vi "Main.vi"() -> ()   [LabVIEW 2013]
uses:
  Global.vi
panel:
  out "Error TCP_quad":errorcluster
  out "TCP_quad ID":refnum<k5>
  in  "Quadcopter":bool
  out "Trailers":bool[](array[boolean])
  out "Platooning Distance Scenario":dbl
  out "Distance2Master Scenario":dbl[](array[numeric])
  out "CurrentWP Final DarkGrey":i32
  out "Vref DarkGrey Final":dbl
  out "CurrentWP Final Grey":i32
  out "Vref Grey Final":dbl
  out "CurrentWP Final Black":i32
  out "Vref Black Final":dbl
  out "CurrentWP Final Blue":i32
  out "Vref Blue Final":dbl
  out "CurrentWP Final Red":i32
  out "Vref Red Final":dbl
  in  "Platooning Speed  Increment":dbl=1.25
  out "StopArrayOuter":i32[](array[numeric])
  out "StopArrayInner":i32[](array[numeric])
  out "PlatoonArray":i32[](array[numeric])
  out "Grey Truck Pose":sgl[](array[numeric])
  out "DarkGrey Truck Pose":dbl[](array[numeric])
  out "Current DarkGrey State":i32
  out "DarkGrey Trajectory WP Out":dbl[][](array[numeric])
  out "Red distance2Master DarkGrey":dbl
  out "DarkGrey dref":dbl
  out "Red distance2Master Grey":dbl
  out "Current Grey State":i32
  out "Grey Trajectory WP Out":dbl[][](array[numeric])
  out "Grey dref":dbl
  out "Change to state DarkGrey Scenario":i32
  out "Vref DarkGrey Scenario":dbl
  out "Change to state Grey Scenario":i32
  out "Vref Grey Scenario":dbl
  in  "ID DarkGrey":u8=5
  in  "ID Grey":u8=4
  in  "Change to state DarkGrey":i32(ring)=1 items=["Parking", "OuterLane", "InnerLane", "InnerRoad"]
  in  "Vref DarkGrey":dbl(slide) scale=0.0..1.5
  in  "Change to state Grey":i32(ring)=1 items=["Parking", "OuterLane", "InnerLane", "InnerRoad"]
  in  "Vref Grey":dbl(slide) scale=0.0..1.5
  out "X Grey":dbl
  out "Y  Grey":dbl
  out "Yaw  Grey":dbl
  out "X DarkGrey":dbl
  out "Y  DarkGrey":dbl
  out "Yaw  DarkGrey":dbl
  in  "ControllerGains DarkGrey":T1={"KPSteering"=1.0, "KDSteering"=0.0, "KPSpeed"=0.8, "KISpeed"=3.0, "KDSpeed"=0.2}
  out "Current state DarkGrey":i32(ring)=1 items=["Parking", "OuterLane", "InnerLane", "InnerRoad"]
  out "D2TL DarkGrey":dbl
  out "D2Master DarkGrey":dbl
  in  "With Trailer DarkGrey":bool
  out "Real Speed DarkGrey":dbl(knob) scale=0.0..2.0
  out "DarkGrey Speed":u8
  out "DarkGrey Steering":u8
  in  "ControllerGains Grey":T1={"KPSteering"=0.6, "KDSteering"=0.05, "KPSpeed"=0.8, "KISpeed"=3.0, "KDSpeed"=0.2}
  out "Current state Grey":i32(ring)=1 items=["Parking", "OuterLane", "InnerLane", "InnerRoad"]
  out "D2TL Grey":dbl
  out "D2Master Grey":dbl
  in  "With Trailer Grey":bool
  out "Real Speed Grey":dbl(knob) scale=0.0..2.0
  out "Grey Speed":u8
  out "Grey Steering":u8
  out "COM  DarkGrey":T2
  out "COM  Grey":T2
  in  "DarkGrey ID":u8=9
  in  "Grey ID":u8=8
  in  "Port DarkGrey":u16=9006
  in  "Port Grey":u16=9005
  in  "QTM ID DarkGrey":i32=3
  in  "QTM ID Grey":i32=5
  out "Vref":dbl[](array[numeric])
  out "bytes written 3":i32
  out "bytes written 2":i32
  out "ScenarioString":string
  out "red dref":dbl
  out "real distance2master red":dbl
  in  "ControllerGains Black":T1={"KPSteering"=0.9, "KDSteering"=0.05, "KPSpeed"=1.0, "KISpeed"=3.0, "KDSpeed"=0.2}
  in  "ControllerGains Blue":T1={"KPSteering"=1.0, "KDSteering"=0.05, "KPSpeed"=0.8, "KISpeed"=3.0, "KDSpeed"=0.2}
  out "Version":i32
  in  "Visualizer":bool
  out "Iter":i32
  out "NRoads":i32
  out "TL Outer Select":bool
  out "TL Inner Select":bool
  out "Error TCP":errorcluster
  out "TCP ID":refnum<k5>
  out "NTrucks":i32
  out "CurrentWP":i32[](array[numeric])
  out "Change to state Red Scenario":i32
  out "Vref Red Scenario":dbl
  out "Change to state Blue Scenario":i32
  out "Vref Blue Scenario":dbl
  out "Change to state Black Scenario":i32
  out "Vref Black Scenario":dbl
  out "Ignore":bool
  out "Current state Red":i32(ring)=1 items=["Parking", "OuterLane", "InnerLane", "InnerRoad"]
  out "Current state Blue":i32(ring)=1 items=["Parking", "OuterLane", "InnerLane", "InnerRoad"]
  out "Current state Black":i32(ring)=1 items=["Parking", "OuterLane", "InnerLane", "InnerRoad"]
  in  "Tab Control":enum32{"Pedro Lima", "João Pedro Alvito"}(tab)
  in  "Scenario Selection PL":u32(ring) items=["Manual", "1 catch up 1", "1 catch up 2", "2 catch up 1", "1 catch up 1 from other road", "1 catch up 1 but master exits", "1 diferent mass catch up 2 without overtake", "1 different mass catch up 2 with overtake", "1 catch up 2 but middle leaves"]
  out "Info PL":string
  out "length":i32
  in  "Bridge":bool
  in  "Scenario Selection JPA":u32(ring) items=["Manual", "Simple traffic lights", "Simple anti-platoon", "Mixture", "Time Decision", "Timed Control with Platoon", "Anti-platoon"]
  out "Info JP":string
  out "X Red":dbl
  out "Y  Red":dbl
  out "Yaw  Red":dbl
  out "X Black":dbl
  out "Y Black":dbl
  out "Yaw Black":dbl
  out "Yaw Blue":dbl
  out "Y Blue":dbl
  out "X Blue":dbl
  out "D2TL Red":dbl
  out "D2TL Black":dbl
  out "D2TL Blue":dbl
  out "D2Master Red":dbl
  out "D2Master Black":dbl
  out "D2Master Blue":dbl
  out "Outer Red":bool
  out "Inner Green":bool
  out "Inner Red":bool
  out "Outer Green":bool
  out "D2TLFinal":dbl[](array[numeric])
  out "Truck Dimensions":dbl[](array[numeric])
  out "Traffic Lights":T3
  in  "Stop Button Inner":bool
  in  "Traffic Light Position Inner Lane":i32=23
  out "CurrentState":i32[](array[numeric])
  out "Real Speed Red":dbl(knob) scale=0.0..2.0
  out "Real Speed Black":dbl(knob) scale=0.0..2.0
  in  "Stop Button Outer":bool
  in  "Traffic Light Position Outer Lane":i32=27
  out "InnerRoad":T4
  out "Distance to Master":dbl[](array[numeric])
  out "Blue dref":dbl
  out "Blue distance2master blue":dbl
  out "black dref":dbl
  out "Red distance2Master black":dbl
  out "Red Trajectory WP Out":dbl[][](array[numeric])
  out "Blue Trajectory WP Out":dbl[][](array[numeric])
  out "Black Trajectory WP Out":dbl[][](array[numeric])
  in  "Change to state Black":i32(ring)=1 items=["Parking", "OuterLane", "InnerLane", "InnerRoad"]
  in  "Change to state Red":i32(ring)=1 items=["Parking", "OuterLane", "InnerLane", "InnerRoad"]
  out "Trajectory Network":T5(array[cluster])
  out "InnerLane":T4
  out "OuterLane":T4
  out "Current Red State":i32
  out "Current Black State":i32
  out "Current Blue State":i32
  in  "Change to state Blue":i32(ring)=1 items=["Parking", "OuterLane", "InnerLane", "InnerRoad"]
  out "Trucks Poses":dbl[][](array[numeric])
  out "Total Platooning Distance":dbl[](array[numeric])
  in  "With Trailer Red":bool
  in  "With Trailer  Black":bool
  in  "With Trailer Blue":bool
  in  "QTM ID Red":i32=4
  in  "QTM ID Blue":i32=2
  in  "QTM ID Black":i32=1
  in  "ID Black":u8=2
  in  "ID Red":u8=3
  in  "ID Blue":u8=1
  out "COM  Black":T2
  out "COM  Red":T2
  out "COM Blue":T2
  in  "Platooning Distance":dbl=0.3
  out "Distance2Master":dbl[](array[numeric])
  out "Real Speed Blue":dbl(knob) scale=0.0..2.0
  in  "Set MasterID":i32(ring) items=["None", "Blue Truck", "Black Truck", "Red Truck", "Grey Truck", "DarkGrey Truck"]
  in  "Vref Black":dbl(slide) scale=0.0..1.5
  in  "Vref Blue":dbl(slide) scale=0.0..1.5
  in  "Vref Red":dbl(slide) scale=0.0..1.5
  out "Red Truck Pose":dbl[](array[numeric])
  out "Blue Truck Pose":dbl[](array[numeric])
  out "Black Truck Pose":dbl[](array[numeric])
  out "Red Speed":u8
  out "Red Steering":u8
  in  "stop":bool
  out "Blue Speed":u8
  out "Blue Steering":u8
  in  "Port Blue":u16=9002
  in  "Blue ID":u8=10
  in  "Port":u16=22222 min=22222
  in  "Address":string="130.237.50.220"
  in  "Port Red":u16=9004
  in  "Red ID":u8=7
  out "Black Speed":u8
  out "Black Steering":u8
  in  "Port Black":u16=9003
  in  "Black ID":u8=14
  in  "ControllerGains Red":T1={"KPSteering"=1.0, "KDSteering"=0.05, "KPSpeed"=0.8, "KISpeed"=3.0, "KDSpeed"=0.2}
types:
  T1 = cluster{"KPSteering":dbl, "KDSteering":dbl, "KPSpeed":dbl, "KISpeed":dbl, "KDSpeed":dbl}
  T2 = cluster{"Truck ID":u8, "connection ID":refnum<k5>}
  T3 = cluster{"Stop Button Outer":bool, "Stop WP Outer Lane":dbl, "Stop Button Inner":bool, "Stop WP Inner Lane ":dbl}
  T4 = cluster{"all rows":dbl[][], "all rows":dbl[][], "Array":i32[]}
  T5 = cluster{"Trajectory WP":dbl[][], "Distances LUT":dbl[][], "Trajectory length":i32[]}[]
  T6 = cluster{"pose":dbl[], "totalerror_v":dbl, "erroSteering":dbl, "ActualTime":dbl, "ActualTime 2":dbl}
  T7 = cluster{"all rows":dbl[][], "all rows":dbl[][], "Array":i32[]}[]
  T8 = cluster{"Trajectory WP":dbl[][], "Distances LUT":dbl[][], "Trajectory length":i32[]}
  T9 = cluster{"Vref Black":dbl, "Change to state Black":i32, "Vref Blue":dbl, "Change to state Blue":i32, "Vref Red":dbl, "Change to state Red":i32, "Vref Grey":dbl, "Change to state Grey":i32, "Vref DarkGrey":dbl, "Change to state DarkGrey":i32, "With Trailer Blue":bool, "With Trailer  Black":bool, "With Trailer Red":bool, "With Trailer Grey":bool, "With Trailer DarkGrey":bool, "Platooning Distance":dbl, "CurrentWP":i32[], "Distance to Master":dbl[], "D2TLFinal":dbl[], "CurrentState":i32[], "Trajectory Network":cluster{"Trajectory WP":dbl[][], "Distances LUT":dbl[][], "Trajectory length":i32[]}[]}
  T10 = cluster{"Vref_Black":dbl, "Change_to_state_Black":i32, "Vref_Blue":dbl, "Change_to_state_Blue":i32, "Vref_Red":dbl, "Change_to_state_Red":i32, "Vref_Grey":dbl, "Change_to_state_Grey":i32, "Vref_DarkGrey":dbl, "Change_to_state_DarkGrey":i32, "With_Trailer_Blue":bool, "With_Trailer_Black":bool, "With_Trailer_Red":bool, "With_Trailer_Grey":bool, "With_Trailer_DarkGrey":bool, "Platooning_Distance":dbl, "CurrentWP":i32[], "Distance2Master":dbl[], "d2TL":dbl[], "CurrentState":i32[], "TrajectoryNetwork":cluster{"TrajectoryWP":dbl[][], "DistancesLUT":dbl[][], "TrajectoryLength":i32[]}[]}
  T11 = cluster{"Stop Button Outer":bool, "Traffic Light Position Outer Lane":i32, "Stop Button Inner":bool, "Traffic Light Position Inner Lane":i32}
  T12 = cluster{"pose":dbl[], "totalerror_v":dbl, "erroSteering":dbl, "ActualTime":dbl, "error_v":dbl}
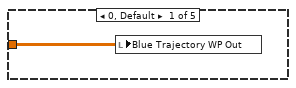
[diagram p5: hidden frame]
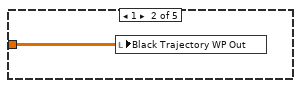
[diagram p6: hidden frame]
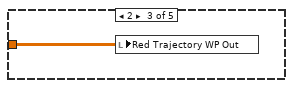
[diagram p7: hidden frame]
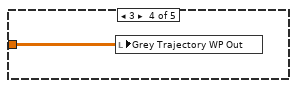
[diagram p8: hidden frame]
diagram:
  n1 = flat-sequence {
    frame #0 {
      n2 = flat-sequence {
        frame #0 {
          # "Initializations"
          n3 = Build Array(0 ("element"), 0 ("element"), 0 ("element"), 0 ("element"), 0 ("element")) -> (w78:i32[])
          "CurrentState" <- w78
          n4 = Build Array(0 ("element"), 0 ("element"), 0 ("element"), 0 ("element"), 0 ("element")) -> (→"CurrentWP":i32[])
          n5 = global write "Global.vi" "Transition WP"(i32[][] [[-1, -1, -1, -1], [-1, -1, -1, -1], [-1, -1, 5, 1], [-1, -1, 50, 25]] ("Transition WP")) -> ()
          n6 = global write "Global.vi" "RealSpeed"(dbl[] [] ("RealSpeed")) -> ()
          n7 = Build Array("Tab Control", "Scenario Selection PL", "Scenario Selection JPA") -> (w59:u32[])
          n8 = global write "Global.vi" "ScenarioArray"(w59) -> ()
          n9 = Array Size(array=w78) -> (size(s)=→"NTrucks":i32)
          n10 = local write "Set MasterID"(0 ("MasterID")) -> ()
          n11 = global write "Global.vi" "IsOvertaking"(FALSE ("IsOvertaking")) -> ()
          n12 = Index Array(array=w59, index=0) -> (element=w60:u32)
          n13 = global write "Global.vi" "Positioned"(FALSE ("FirstTime")) -> ()
          n14 = global write "Global.vi" "MasterID"(0 ("MasterID")) -> ()
          n15 = Increment(x=w60) -> (x+1=w61:u32)
          n16 = global write "Global.vi" "stop"(FALSE ("stop")) -> ()
          n17 = Index Array(array=w59, index=w61) -> (element=w62:u32)
          n18 = global write "Global.vi" "TL  Inner"(FALSE ("TL  Inner")) -> ()
          n19 = global write "Global.vi" "TL Outer"(FALSE ("TL Outer")) -> ()
          n20 = global write "Global.vi" "Lap Counter"(0 ("Lap Counter")) -> ()
          n21 = global write "Global.vi" "FirstTime"(TRUE ("FirstTime")) -> ()
          n22 = Not Equal To 0?(x=w62) -> (x != 0?=→"Ignore":bool)
          n23 = global write "Global.vi" "SetMasterID"(0 ("MasterID")) -> ()
          "ScenarioString" <- " " ("ScenarioString")
          "Vref" <- dbl[] [] ("RealSpeed")
        }
      }
      n24 = flat-sequence {
        frame #0 {
          n25 = local read "Tab Control"() -> (w2:enum32{"Pedro Lima", "João Pedro Alvito"})
          n26 = call "GetVersion.vi"() -> ("number"=→"Version":i32)
          n27 = Not Equal To 0?(x=w2) -> (x != 0?=w1:bool)
          n28 = local read "Version"() -> (w7:i32)
          n29 = local read "Version"() -> (w8:i32)
          n30 = local read "Version"() -> (w9:i32)
          n31 = local read "Version"() -> (w10:i32)
          n32 = local read "Version"() -> (w12:i32)
          n33 = local read "Version"() -> (w14:i32)
          n34 = local read "Version"() -> (w6:i32)
          n35 = local read "Version"() -> (w13:i32)
          n36 = call "CreatePath.vi"("Matlab Version"=w7, "filename"="OuterLaneBridgeLUT.txt") -> ("FinalPath"=w20:path)
          n37 = call "CreatePath.vi"("Matlab Version"=w8, "filename"="OuterLaneLUT.txt") -> ("FinalPath"=w22:path)
          n38 = call "CreatePath.vi"("Matlab Version"=w9, "filename"="OuterLaneBridge.txt") -> ("FinalPath"=w24:path)
          n39 = call "CreatePath.vi"("Matlab Version"=w10, "filename"="OuterLane.txt") -> ("FinalPath"=w26:path)
          n40 = call "CreatePath.vi"("Matlab Version"=w12, "filename"="InnerLaneBridgeLUT.txt") -> ("FinalPath"=w34:path)
          n41 = call "CreatePath.vi"("Matlab Version"=w14, "filename"="InnerLaneLUT.txt") -> ("FinalPath"=w33:path)
          n42 = call "CreatePath.vi"("Matlab Version"=w6, "filename"="InnerLaneBridge.txt") -> ("FinalPath"=w30:path)
          n43 = call "CreatePath.vi"("Matlab Version"=w13, "filename"="InnerLane.txt") -> ("FinalPath"=w28:path)
          n44 = local read "Version"() -> (w11:i32)
          n45 = local read "Version"() -> (w15:i32)
          n46 = And(x="Bridge", y=w1) -> (x .and. y?=w4:bool)
          n47 = call "CreatePath.vi"("Matlab Version"=w11, "filename"="InnerRoadLUT.txt") -> ("FinalPath"=w16:path)
          n48 = call "CreatePath.vi"("Matlab Version"=w15, "filename"="InnerRoad.txt") -> ("FinalPath"=w18:path)
          n49 = Select(t=w20, s=w4, f=w22) -> (s? t:f=w41:path)
          n50 = Select(t=w24, s=w4, f=w26) -> (s? t:f=w40:path)
          n51 = Select(t=w34, s=w4, f=w33) -> (s? t:f=w38:path)
          n52 = Select(t=w30, s=w4, f=w28) -> (s? t:f=w39:path)
          n53 = call "ReadFromFile.vi"("Trajectory Path File"=w40, "Trajectory Distances LUT"=w41) -> ("Trajectory Data"=w45:T4)  [unwired: 1 in]
          "OuterLane" <- w45
          n54 = call "ReadFromFile.vi"("Trajectory Path File"=w18, "Trajectory Distances LUT"=w16) -> ("Trajectory Data"=w42:T4)  [unwired: 1 in]
          "InnerRoad" <- w42
          n55 = call "ReadFromFile.vi"("Trajectory Path File"=w39, "Trajectory Distances LUT"=w38) -> ("Trajectory Data"=w44:T4)  [unwired: 1 in]
          "InnerLane" <- w44
          n56 = Build Array(T4 {"all rows"=[], "all rows"=[], "Array"=[]} ("element"), w45, w44, w42) -> (w37:T7)
          "Trajectory Network" <- w37
          n57 = Array Size(array=w37) -> (size(s)=→"NRoads":i32)
        }
      }
      n58 = flat-sequence {
        frame #0 {
          n59 = call "CreateConnection.vi"("Truck ID"="DarkGrey ID", "Port number\nactuators"="Port DarkGrey") -> ("COM data"=→"COM  DarkGrey":T2)  [unwired: 1 in]
          n60 = call "CreateConnection.vi"("Truck ID"="Red ID", "Port number\nactuators"="Port Red") -> ("COM data"=→"COM  Red":T2)  [unwired: 1 in]
          n61 = call "CreateConnection.vi"("Truck ID"="Black ID", "Port number\nactuators"="Port Black") -> ("COM data"=→"COM  Black":T2)  [unwired: 1 in]
          n62 = call "CreateConnection.vi"("Truck ID"="Blue ID", "Port number\nactuators"="Port Blue") -> ("COM data"=→"COM Blue":T2)  [unwired: 1 in]
          n63 = call "CreateConnection.vi"("Truck ID"="Grey ID", "Port number\nactuators"="Port Grey") -> ("COM data"=→"COM  Grey":T2)  [unwired: 1 in]
        }
      }
    }
    frame #1 {
      n64 = local read "Visualizer"() -> (w98:bool)
      n65 = local read "Quadcopter"() -> (w97:bool)
      n66 = case shown="True" w98 {
        frame False {
        }
        frame True {
          n67 = flat-sequence {
            frame #0 {
              n68 = local read "Trajectory Network"() -> (w109:T5)
              n69 = Index Array(array=w109) -> (element #2=w110:T8, element #3=w111:T8, element #4=w112:T8)  [unwired: 4 in, 1 out]
              n70 = Unbundle By Name(w110) -> ("Trajectory length"=w116:i32[], "Trajectory WP"=w124:dbl[][])
              n71 = Unbundle By Name(w111) -> ("Trajectory length"=w120:i32[], "Trajectory WP"=w125:dbl[][])
              n72 = Unbundle By Name(w112) -> ("Trajectory length"=w121:i32[], "Trajectory WP"=w126:dbl[][])
              n73 = Index Array(array=w116, index=0) -> (element=w127:i32)
              n74 = Index Array(array=w120, index=0) -> (element=w129:i32)
              n75 = Index Array(array=w121, index=0) -> (element=w131:i32)
              n76 = local read "NRoads"() -> (w138:i32)
              n77 = Multiply(x=w127, y=2) -> (x*y=w122:i32)
              n78 = Multiply(x=w129, y=2) -> (x*y=w123:i32)
              n79 = Multiply(x=w131, y=2) -> (x*y=w103:i32)
              n80 = Reshape Array(w124, w122) -> (w128:dbl[])
              n81 = Reshape Array(w125, w123) -> (w130:dbl[])
              n82 = Reshape Array(w126, w103) -> (w132:dbl[])
              n83 = Subtract(x=w138, y=1) -> (x-y=w139:i32)
              n84 = Build Array (concatenate)(w139, w127, w128, w129, w130, w131, w132) -> (w106:dbl[])
              n85 = To Double Precision Float(number=w106) -> (double precision float=w107:dbl[])
              n86 = Type Cast(x=w107) -> (*(type *) &x=w108:string)  [unwired: 1 in]
              n87 = call <vilib>:"TCP Listen.vi"("timeout ms (wait forever: -1)"=-1, "port"=u16 55000 ("remote port or service name")) -> ("error out"=w134:errorcluster, "connection ID"=w133:refnum<k5>)  [unwired: 5 in, 3 out]
              n88 = TCP Write(connection ID=w133, data in=w108, error in (no error)=w134) -> (connection ID out=→"TCP ID":refnum<k5>, error out=→"Error TCP":errorcluster)  [unwired: 1 in, 1 out]
            }
            frame #1 {
              n89 = local read "Bridge"() -> (w141:bool)
              n90 = Boolean To (0,1)(Boolean=w141) -> (0, 1=w140:i16)
              n91 = global read "Global.vi" "ScenarioArray"() -> (w143:u32[])
              n92 = local read "NTrucks"() -> (w142:i32)
              n93 = Build Array (concatenate)(w143, w142, w140) -> (w145:u32[])
              n94 = To Double Precision Float(number=w145) -> (double precision float=w144:dbl[])
              n95 = Type Cast(x=w144) -> (*(type *) &x=w146:string)  [unwired: 1 in]
              n96 = local read "Error TCP"() -> (w148:errorcluster)
              n97 = local read "TCP ID"() -> (w147:refnum<k5>)
              n98 = TCP Write(connection ID=w147, data in=w146, error in (no error)=w148) -> (connection ID out=w150:refnum<k5>, error out=w149:errorcluster)  [unwired: 1 in, 1 out]
              n99 = local write "TCP ID"(w150) -> ()
              n100 = local write "Error TCP"(w149) -> ()
            }
          }
        }
      }
      n101 = case shown="True" w97 {
        frame False {
        }
        frame True {
          n102 = call <vilib>:"TCP Listen.vi"("timeout ms (wait forever: -1)"=-1, "port"=u16 56999 ("remote port or service name")) -> ("error out"=→"Error TCP_quad":errorcluster, "connection ID"=→"TCP_quad ID":refnum<k5>)  [unwired: 5 in, 3 out]
        }
      }
    }
    frame #2 {
      n103 = while {
        i -> [w151]
        stop <- "stop" stop-if-true
        n104 = flat-sequence {
          frame #0 {
            n105 = call "GetPose.vi"("port"="Port", "address"="Address", "QTM ID"="QTM ID Blue") -> ("Pose"=w164:dbl[])  [unwired: 8 in]
            "Blue Truck Pose" <- w164
            n106 = call "GetPose.vi"("port"="Port", "address"="Address", "QTM ID"="QTM ID Grey") -> ("Pose"=w160:dbl[])  [unwired: 8 in]
            "Grey Truck Pose" <- w160
            n107 = call "GetPose.vi"("port"="Port", "address"="Address", "QTM ID"="QTM ID DarkGrey") -> ("Pose"=w158:dbl[])  [unwired: 8 in]
            "DarkGrey Truck Pose" <- w158
            n108 = call "GetPose.vi"("port"="Port", "address"="Address", "QTM ID"="QTM ID Black") -> ("Pose"=w162:dbl[])  [unwired: 8 in]
            "Black Truck Pose" <- w162
            n109 = call "GetPose.vi"("port"="Port", "address"="Address", "QTM ID"="QTM ID Red") -> ("Pose"=w156:dbl[])  [unwired: 8 in]
            "Red Truck Pose" <- w156
            n110 = Build Array(w164, w162, w156, w160, w158) -> (→"Trucks Poses":dbl[][])
            n111 = Index Array(array=w164) -> (element #1=→"X Blue":dbl, element #2=→"Y Blue":dbl, element #3=→"Yaw Blue":dbl)  [unwired: 3 in]
            n112 = Index Array(array=w162) -> (element #1=→"X Black":dbl, element #2=→"Y Black":dbl, element #3=→"Yaw Black":dbl)  [unwired: 3 in]
            n113 = Index Array(array=w160) -> (element #1=→"X Grey":dbl, element #2=→"Y  Grey":dbl, element #3=→"Yaw  Grey":dbl)  [unwired: 3 in]
            n114 = Index Array(array=w158) -> (element #1=→"X DarkGrey":dbl, element #2=→"Y  DarkGrey":dbl, element #3=→"Yaw  DarkGrey":dbl)  [unwired: 3 in]
            n115 = Index Array(array=w156) -> (element #1=→"X Red":dbl, element #2=→"Y  Red":dbl, element #3=→"Yaw  Red":dbl)  [unwired: 3 in]
          }
          frame #1 {
            w193 = 0.5 ("t")
            w194 = 1.3 ("t")
            n116 = local read "Trajectory Network"() -> (w207:T5)
            n117 = local read "Distance to Master"() -> (w210:dbl[])
            n118 = local read "CurrentState"() -> (w208:i32[])
            n119 = local read "CurrentWP"() -> (w211:i32[])
            n120 = local read "D2TLFinal"() -> (w209:dbl[])
            n121 = Bundle("Vref Black"="Vref Black", "Change to state Black"="Change to state Black", "Vref Blue"="Vref Blue", "Change to state Blue"="Change to state Blue", "Vref Red"="Vref Red", "Change to state Red"="Change to state Red", "Vref Grey"="Vref Grey", "Change to state Grey"="Change to state Grey", "Vref DarkGrey"="Vref DarkGrey", "Change to state DarkGrey"="Change to state DarkGrey", "With Trailer Blue"="With Trailer Blue", "With Trailer  Black"="With Trailer  Black", "With Trailer Red"="With Trailer Red", "With Trailer Grey"="With Trailer Grey", "With Trailer DarkGrey"="With Trailer DarkGrey", "Platooning Distance"="Platooning Distance", "CurrentWP"=w211, "Distance to Master"=w210, "D2TLFinal"=w209, "CurrentState"=w208, "Trajectory Network"=w207) -> (w199:T9)  [unwired: 1 in]
            n122 = call "ScenarioScript.vi"("Control In"=w199) -> ("Control Out"=w219:T10, "String"=w206:string)
            "Info PL" <- w206
            "Info JP" <- w206
            n123 = local write "ScenarioString"(w206) -> ()
            n124 = Unbundle By Name(w219) -> ("Vref_Black"=→"Vref Black Scenario":dbl, "Change_to_state_Black"=→"Change to state Black Scenario":i32, "Vref_Blue"=→"Vref Blue Scenario":dbl, "Change_to_state_Blue"=→"Change to state Blue Scenario":i32, "Vref_Red"=→"Vref Red Scenario":dbl, "Change_to_state_Red"=→"Change to state Red Scenario":i32, "Vref_Grey"=→"Vref Grey Scenario":dbl, "Change_to_state_Grey"=→"Change to state Grey Scenario":i32, "Vref_DarkGrey"=→"Vref DarkGrey Scenario":dbl, "Change_to_state_DarkGrey"=→"Change to state DarkGrey Scenario":i32, "With_Trailer_Blue"=w187:bool, "With_Trailer_Black"=w186:bool, "With_Trailer_Red"=w185:bool, "With_Trailer_Grey"=w184:bool, "With_Trailer_DarkGrey"=w183:bool, "Platooning_Distance"=w213:dbl, "Distance2Master"=w190:dbl[])
            "Platooning Distance Scenario" <- w213
            n125 = Select(t=w194, s=w187, f=w193) -> (s? t:f=w230:dbl)
            n126 = Select(t=w194, s=w186, f=w193) -> (s? t:f=w231:dbl)
            n127 = Select(t=w194, s=w185, f=w193) -> (s? t:f=w232:dbl)
            n128 = Select(t=w194, s=w184, f=w193) -> (s? t:f=w192:dbl)
            n129 = Select(t=w194, s=w183, f=w193) -> (s? t:f=w191:dbl)
            n130 = Build Array(w187, w186, w185, w184, w183) -> (→"Trailers":bool[])
            n131 = Build Array(w230, w231, w232, w192, w191) -> (w189:dbl[])
            "Truck Dimensions" <- w189
            n132 = Add(x=w189, y=w213) -> (x+y=→"Total Platooning Distance":dbl[])
            n133 = Add(x=w190, y=w189) -> (x+y=→"Distance2Master Scenario":dbl[])
          }
          frame #2 {
            n134 = local read "Change to state DarkGrey Scenario"() -> (w281:i32)
            n135 = local read "Change to state Black Scenario"() -> (w304:i32)
            n136 = local read "Change to state Grey Scenario"() -> (w294:i32)
            n137 = local read "Change to state Blue Scenario"() -> (w303:i32)
            n138 = local read "Platooning Speed  Increment"() -> (w264:dbl)
            n139 = local read "Platooning Speed  Increment"() -> (w268:dbl)
            n140 = local read "Platooning Speed  Increment"() -> (w267:dbl)
            n141 = local read "Change to state Red Scenario"() -> (w305:i32)
            n142 = local read "Platooning Speed  Increment"() -> (w266:dbl)
            n143 = local read "Platooning Speed  Increment"() -> (w265:dbl)
            n144 = local read "Total Platooning Distance"() -> (w314:dbl[])
            n145 = local read "Distance2Master Scenario"() -> (w328:dbl[])
            n146 = local read "Total Platooning Distance"() -> (w290:dbl[])
            n147 = local read "Distance2Master Scenario"() -> (w286:dbl[])
            n148 = local read "Total Platooning Distance"() -> (w277:dbl[])
            n149 = local read "Distance2Master Scenario"() -> (w273:dbl[])
            n150 = local read "Total Platooning Distance"() -> (w330:dbl[])
            n151 = local read "Distance2Master Scenario"() -> (w329:dbl[])
            n152 = local read "Total Platooning Distance"() -> (w318:dbl[])
            n153 = local read "Distance2Master Scenario"() -> (w319:dbl[])
            n154 = local read "Vref DarkGrey Scenario"() -> (w254:dbl)
            n155 = local read "Real Speed DarkGrey"() -> (w269:dbl)
            n156 = local read "Trajectory Network"() -> (w316:T5)
            n157 = local read "Trajectory Network"() -> (w288:T5)
            n158 = local read "Trajectory Network"() -> (w275:T5)
            n159 = local read "Trajectory Network"() -> (w335:T5)
            n160 = local read "Trajectory Network"() -> (w321:T5)
            n161 = local read "Vref Black Scenario"() -> (w256:dbl)
            n162 = local read "Vref Grey Scenario"() -> (w255:dbl)
            n163 = local read "Vref Red Scenario"() -> (w258:dbl)
            n164 = local read "Vref Blue Scenario"() -> (w257:dbl)
            n165 = local read "Real Speed Black"() -> (w327:dbl)
            n166 = local read "Real Speed Blue"() -> (w339:dbl)
            n167 = local read "Real Speed Grey"() -> (w270:dbl)
            n168 = local read "Real Speed Red"() -> (w326:dbl)
            n169 = local read "PlatoonArray"() -> (w236:i32[])
            n170 = local read "Traffic Lights"() -> (w322:T3)
            n171 = local read "PlatoonArray"() -> (w235:i32[])
            n172 = local read "Traffic Lights"() -> (w287:T3)
            n173 = local read "PlatoonArray"() -> (w234:i32[])
            n174 = local read "Traffic Lights"() -> (w274:T3)
            n175 = local read "PlatoonArray"() -> (w238:i32[])
            n176 = local read "Traffic Lights"() -> (w323:T3)
            n177 = local read "PlatoonArray"() -> (w237:i32[])
            n178 = local read "Traffic Lights"() -> (w324:T3)
            n179 = local read "Trucks Poses"() -> (w315:dbl[][])
            n180 = local read "Trucks Poses"() -> (w289:dbl[][])
            n181 = local read "Trucks Poses"() -> (w276:dbl[][])
            n182 = local read "Trucks Poses"() -> (w333:dbl[][])
            n183 = local read "Trucks Poses"() -> (w331:dbl[][])
            n184 = local read "CurrentState"() -> (w312:i32[])
            n185 = local read "Set MasterID"() -> (w261:i32)
            n186 = local read "CurrentState"() -> (w292:i32[])
            n187 = local read "Set MasterID"() -> (w262:i32)
            n188 = local read "CurrentState"() -> (w279:i32[])
            n189 = local read "Set MasterID"() -> (w263:i32)
            n190 = local read "CurrentState"() -> (w325:i32[])
            n191 = local read "Set MasterID"() -> (w259:i32)
            n192 = local read "CurrentState"() -> (w317:i32[])
            n193 = local read "Set MasterID"() -> (w260:i32)
            n194 = local read "ID DarkGrey"() -> (w278:u8)
            n195 = local read "CurrentWP"() -> (w251:i32[])
            n196 = local read "CurrentWP"() -> (w250:i32[])
            n197 = local read "CurrentWP"() -> (w249:i32[])
            n198 = local read "CurrentWP"() -> (w253:i32[])
            n199 = local read "CurrentWP"() -> (w252:i32[])
            n200 = local read "D2TLFinal"() -> (w309:dbl[])
            n201 = local read "D2TLFinal"() -> (w293:dbl[])
            n202 = local read "D2TLFinal"() -> (w280:dbl[])
            n203 = local read "D2TLFinal"() -> (w311:dbl[])
            n204 = local read "D2TLFinal"() -> (w310:dbl[])
            n205 = local read "ID Black"() -> (w313:u8)
            n206 = local read "ID Grey"() -> (w291:u8)
            n207 = local read "ID Blue"() -> (w320:u8)
            n208 = local read "ID Red"() -> (w334:u8)
            n209 = call "DecisionMaker.vi"("Trajectory Network"=w316, "Change to state"=w304, "Vref"=w256, "K"=w264, "Platooning distances"=w314, "Current State In"=w312, "Set MasterID"=w261, "Current WP In"=w251, "MyID"=w313, "Distance2Master"=w328, "PlatoonArray"=w236, "Traffic Lights"=w322, "Trucks Poses"=w315, "d2TLFinal"=w309) -> ("d"=→"Red distance2Master black":dbl, "dref"=→"black dref":dbl, "Current State Out"=→"Current Black State" →"Current state Black":i32, "VrefOut"=→"Vref Black Final":dbl, "CurrentWPOut"=→"CurrentWP Final Black":i32, "Trajectory WP Out"=→"Black Trajectory WP Out":dbl[][])  [unwired: 8 in]
            n210 = call "DecisionMaker.vi"("Trajectory Network"=w288, "Change to state"=w294, "Vref"=w255, "K"=w268, "Platooning distances"=w290, "Current State In"=w292, "Set MasterID"=w262, "Current WP In"=w250, "MyID"=w291, "Distance2Master"=w286, "PlatoonArray"=w235, "Traffic Lights"=w287, "Trucks Poses"=w289, "d2TLFinal"=w293) -> ("d"=→"Red distance2Master Grey":dbl, "dref"=→"Grey dref":dbl, "Current State Out"=→"Current Grey State" →"Current state Grey":i32, "VrefOut"=→"Vref Grey Final":dbl, "CurrentWPOut"=→"CurrentWP Final Grey":i32, "Trajectory WP Out"=→"Grey Trajectory WP Out":dbl[][])  [unwired: 8 in]
            n211 = call "DecisionMaker.vi"("Trajectory Network"=w275, "Change to state"=w281, "Vref"=w254, "K"=w267, "Platooning distances"=w277, "Current State In"=w279, "Set MasterID"=w263, "Current WP In"=w249, "MyID"=w278, "Distance2Master"=w273, "PlatoonArray"=w234, "Traffic Lights"=w274, "Trucks Poses"=w276, "d2TLFinal"=w280) -> ("d"=→"Red distance2Master DarkGrey":dbl, "dref"=→"DarkGrey dref":dbl, "Current State Out"=→"Current state DarkGrey" →"Current DarkGrey State":i32, "VrefOut"=→"Vref DarkGrey Final":dbl, "CurrentWPOut"=→"CurrentWP Final DarkGrey":i32, "Trajectory WP Out"=→"DarkGrey Trajectory WP Out":dbl[][])  [unwired: 8 in]
            n212 = call "DecisionMaker.vi"("Trajectory Network"=w335, "Change to state"=w305, "Vref"=w258, "K"=w266, "Platooning distances"=w330, "Current State In"=w325, "Set MasterID"=w259, "Current WP In"=w253, "MyID"=w334, "Distance2Master"=w329, "PlatoonArray"=w238, "Traffic Lights"=w323, "Trucks Poses"=w333, "d2TLFinal"=w311) -> ("d"=→"real distance2master red":dbl, "dref"=→"red dref":dbl, "Current State Out"=→"Current Red State" →"Current state Red":i32, "VrefOut"=→"Vref Red Final":dbl, "CurrentWPOut"=→"CurrentWP Final Red":i32, "Trajectory WP Out"=→"Red Trajectory WP Out":dbl[][])  [unwired: 8 in]
            n213 = call "DecisionMaker.vi"("Trajectory Network"=w321, "Change to state"=w303, "Vref"=w257, "K"=w265, "Platooning distances"=w318, "Current State In"=w317, "Set MasterID"=w260, "Current WP In"=w252, "MyID"=w320, "Distance2Master"=w319, "PlatoonArray"=w237, "Traffic Lights"=w324, "Trucks Poses"=w331, "d2TLFinal"=w310) -> ("d"=→"Blue distance2master blue":dbl, "dref"=→"Blue dref":dbl, "Current State Out"=→"Current Blue State" →"Current state Blue":i32, "VrefOut"=→"Vref Blue Final":dbl, "CurrentWPOut"=→"CurrentWP Final Blue":i32, "Trajectory WP Out"=→"Blue Trajectory WP Out":dbl[][])  [unwired: 8 in]
            n214 = Build Array(w339, w327, w326, w270, w269) -> (w332:dbl[])
            n215 = global write "Global.vi" "RealSpeed"(w332) -> ()
          }
          frame #3 {
            n216 = flat-sequence {
              frame #0 {
                n217 = local read "CurrentWP Final DarkGrey"() -> (w368:i32)
                n218 = local read "Current DarkGrey State"() -> (w353:i32)
                n219 = local read "CurrentWP Final Black"() -> (w366:i32)
                n220 = local read "CurrentWP Final Blue"() -> (w365:i32)
                n221 = local read "CurrentWP Final Grey"() -> (w369:i32)
                n222 = local read "CurrentWP Final Red"() -> (w367:i32)
                n223 = local read "Current Black State"() -> (w355:i32)
                n224 = local read "Vref DarkGrey Final"() -> (w359:dbl)
                n225 = local read "Current Grey State"() -> (w352:i32)
                n226 = local read "Current Blue State"() -> (w356:i32)
                n227 = local read "Current Red State"() -> (w354:i32)
                n228 = local read "Vref Black Final"() -> (w361:dbl)
                n229 = local read "Vref Grey Final"() -> (w358:dbl)
                n230 = local read "Vref Blue Final"() -> (w362:dbl)
                n231 = local read "Vref Red Final"() -> (w360:dbl)
                n232 = Build Array(w356, w355, w354, w352, w353) -> (w357:i32[])
                n233 = Build Array(w365, w366, w367, w369, w368) -> (w364:i32[])
                n234 = Build Array(w362, w361, w360, w358, w359) -> (w363:dbl[])
                n235 = local write "CurrentState"(w357) -> ()
                n236 = local write "CurrentWP"(w364) -> ()
                n237 = local write "Vref"(w363) -> ()
              }
              frame #1 {
                n238 = global read "Global.vi" "SetMasterID"() -> (w373:i32)
                n239 = local read "Ignore"() -> (w374:bool)
                n240 = Select(t=w373, s=w374, f="Set MasterID") -> (s? t:f=w370:i32)
                n241 = local write "Set MasterID"(w370) -> ()
                n242 = case shown="1, Default" w370 {
                  selector: w370 -> [w375 w380]
                  tunnel: [w375 w379] -> w371
                  frame 0 {
                  }
                  frame 1, Default {
                    n243 = local read "Total Platooning Distance"() -> (w376:dbl[])
                    n244 = local read "Trajectory Network"() -> (w382:T5)
                    n245 = local read "PlatoonArray"() -> (w384:i32[])
                    n246 = local read "Trucks Poses"() -> (w383:dbl[][])
                    n247 = local read "CurrentState"() -> (w381:i32[])
                    n248 = local read "CurrentWP"() -> (w378:i32[])
                    n249 = local read "Vref"() -> (w385:dbl[])
                    n250 = call "OvertakingDecisor.vi"("Trajectory Network"=w382, "PlatoonArray"=w384, "Trucks Poses"=w383, "Current State In"=w381, "Total Platooning Distance"=w376, "Set MasterID"=w380, "CurrentWP"=w378, "Vref"=w385) -> ("VrefOut"=w391:dbl, "Current WP Out"=w390:i32, "Set MasterID Out"=w379:i32, "Current State Out"=w389:i32, "Trajectory WP Out"=w395:dbl[][])  [unwired: 3 in]
                    n251 = Decrement(x=w380) -> (x-1=w394:i32)
                    n252 = local read "CurrentState"() -> (w388:i32[])
                    n253 = case shown="4" w394 {
                      tunnel: w395 -> [w396 w397 w398 w399 w400]
                      frame 0, Default {
                        n254 = local write "Blue Trajectory WP Out"(w396) -> ()
                      }
                      frame 1 {
                        n255 = local write "Black Trajectory WP Out"(w397) -> ()
                      }
                      frame 2 {
                        n256 = local write "Red Trajectory WP Out"(w398) -> ()
                      }
                      frame 3 {
                        n257 = local write "Grey Trajectory WP Out"(w399) -> ()
                      }
                      frame 4 {
                        n258 = local write "DarkGrey Trajectory WP Out"(w400) -> ()
                      }
                    }
                    n259 = local read "CurrentWP"() -> (w386:i32[])
                    n260 = local read "Vref"() -> (w387:dbl[])
                    n261 = Replace Array Subset(array=w387, new element=w391, index=w394) -> (w392:dbl[])
                    n262 = Replace Array Subset(array=w386, new element=w390, index=w394) -> (w393:i32[])
                    n263 = Replace Array Subset(array=w388, new element=w389, index=w394) -> (w377:i32[])
                    n264 = local write "Vref"(w392) -> ()
                    n265 = local write "CurrentWP"(w393) -> ()
                    n266 = local write "CurrentState"(w377) -> ()
                  }
                }
                n267 = global write "Global.vi" "MasterID"(w371) -> ()
              }
            }
            n268 = global read "Global.vi" "TL Outer"() -> (w346:bool)
            n269 = global read "Global.vi" "TL  Inner"() -> (w344:bool)
            n270 = local read "Ignore"() -> (w342:bool)
            n271 = Select(t=w346, s=w342, f="Stop Button Outer") -> (s? t:f=w340:bool)
            "Outer Red" <- w340
            "TL Outer Select" <- w340
            n272 = Select(t=w344, s=w342, f="Stop Button Inner") -> (s? t:f=w341:bool)
            "Inner Red" <- w341
            "TL Inner Select" <- w341
            n273 = Bundle("Stop Button Outer"=w340, "Traffic Light Position Outer Lane"="Traffic Light Position Outer Lane", "Stop Button Inner"=w341, "Traffic Light Position Inner Lane"="Traffic Light Position Inner Lane") -> (→"Traffic Lights":T11)  [unwired: 1 in]
            n274 = Not(x=w340) -> (.not. x?=→"Outer Green":bool)
            n275 = Not(x=w341) -> (.not. x?=→"Inner Green":bool)
          }
          frame #4 {
            n276 = local read "Trajectory Network"() -> (w420:T5)
            n277 = local read "Truck Dimensions"() -> (w418:dbl[])
            n278 = local read "Traffic Lights"() -> (w419:T3)
            n279 = local read "Trucks Poses"() -> (w421:dbl[][])
            n280 = local read "CurrentState"() -> (w422:i32[])
            n281 = local read "CurrentWP"() -> (w409:i32[])
            n282 = global read "Global.vi" "MasterID"() -> (w426:i32)
            n283 = local read "Trajectory Network"() -> (w430:T5)
            n284 = call "GetDistance2TL.vi"("Traffic Lights"=w419, "Truck Dimensions"=w418, "Trajectory Network"=w420, "CurrentWP"=w409, "Trucks Poses"=w421, "Current State"=w422) -> ("StopArray_2"=→"StopArrayInner":i32[], "d2TLFinal"=w413:dbl[], "StopArray_1"=→"StopArrayOuter":i32[])
            "D2TLFinal" <- w413
            n285 = local read "Trucks Poses"() -> (w423:dbl[][])
            n286 = local read "Set MasterID"() -> (w401:i32)
            n287 = Subtract(x=w426, y=1) -> (x-y=w429:i32)
            n288 = local read "Truck Dimensions"() -> (w425:dbl[])
            n289 = local read "CurrentState"() -> (w431:i32[])
            n290 = call "GetDistance2Master.vi"("TrucksPoses"=w423, "Set MasterID"=w401, "Trajectory Network"=w430, "Current State"=w431) -> ("Distance2Master"=w424:dbl[], "PlatoonArray"=→"PlatoonArray":i32[])
            "Distance2Master" <- w424
            n291 = Index Array(array=w425, index=w429) -> (element=w427:dbl)
            n292 = Index Array(array=w413) -> (element #1=→"D2TL Blue":dbl, element #2=→"D2TL Black":dbl, element #3=→"D2TL Red":dbl, element #4=→"D2TL Grey":dbl, element #5=→"D2TL DarkGrey":dbl)  [unwired: 5 in]
            n293 = Subtract(x=w424, y=w427) -> (x-y=w417:dbl[])
            "Distance to Master" <- w417
            n294 = Index Array(array=w417) -> (element #1=→"D2Master Blue":dbl, element #2=→"D2Master Black":dbl, element #3=→"D2Master Red":dbl, element #4=→"D2Master Grey":dbl, element #5=→"D2Master DarkGrey":dbl)  [unwired: 5 in]
          }
          frame #5 {
            n295 = local read "DarkGrey Trajectory WP Out"() -> (w456:dbl[][])
            n296 = local read "Black Trajectory WP Out"() -> (w480:dbl[][])
            n297 = local read "Blue Trajectory WP Out"() -> (w489:dbl[][])
            n298 = local read "Grey Trajectory WP Out"() -> (w469:dbl[][])
            n299 = local read "Red Trajectory WP Out"() -> (w495:dbl[][])
            n300 = local read "DarkGrey Truck Pose"() -> (w460:dbl[])
            n301 = local read "Black Truck Pose"() -> (w505:dbl[])
            n302 = local read "Grey Truck Pose"() -> (w461:sgl[])
            n303 = local read "Blue Truck Pose"() -> (w491:dbl[])
            n304 = local read "Red Truck Pose"() -> (w501:dbl[])
            n305 = local read "CurrentState"() -> (w482:i32[])
            n306 = local read "CurrentState"() -> (w483:i32[])
            n307 = local read "CurrentState"() -> (w481:i32[])
            n308 = local read "CurrentState"() -> (w472:i32[])
            n309 = local read "CurrentState"() -> (w453:i32[])
            n310 = local read "ID DarkGrey"() -> (w457:u8)
            n311 = local read "CurrentWP"() -> (w488:i32[])
            n312 = local read "CurrentWP"() -> (w494:i32[])
            n313 = local read "CurrentWP"() -> (w493:i32[])
            n314 = local read "CurrentWP"() -> (w470:i32[])
            n315 = local read "CurrentWP"() -> (w455:i32[])
            n316 = local read "ID Black"() -> (w507:u8)
            n317 = local read "ID Blue"() -> (w492:u8)
            n318 = local read "ID Grey"() -> (w468:u8)
            n319 = local read "ID Red"() -> (w496:u8)
            n320 = local read "Vref"() -> (w486:dbl[])
            n321 = local read "Vref"() -> (w485:dbl[])
            n322 = local read "Vref"() -> (w487:dbl[])
            n323 = local read "Vref"() -> (w471:dbl[])
            n324 = local read "Vref"() -> (w454:dbl[])
            n325 = Tick Count (ms)() -> (millisecond timer value=w490:u32)
            n326 = Tick Count (ms)() -> (millisecond timer value=w506:u32)
            n327 = Tick Count (ms)() -> (millisecond timer value=w497:u32)
            n328 = Tick Count (ms)() -> (millisecond timer value=w463:u32)
            n329 = Tick Count (ms)() -> (millisecond timer value=w459:u32)
            n330 = local read "COM  DarkGrey"() -> (w446:T2)
            n331 = local read "COM  Black"() -> (w438:T2)
            n332 = local read "COM  Grey"() -> (w466:T2)
            n333 = local read "COM Blue"() -> (w508:T2)
            n334 = local read "COM  Red"() -> (w442:T2)
            n335 = feedback #1(T6 {"pose"=[0.0, 0.0, 0.0], "totalerror_v"=0.0, "erroSteering"=0.0, "ActualTime"=0.0, "ActualTime 2"=0.0} ("Red feedback init")) -> (w432:T6)
            n336 = call "Controller.vi"("ControllerGains"="ControllerGains Blue", "Current State"=w482, "MyID"=w492, "Pose"=w491, "Feedback elements In"=w432, "CurrentWP"=w488, "Vref"=w486, "Trajectory"=w489, "ActualTime"=w490) -> ("Feedback elements Out"=w433:T12, "v_real"=→"Real Speed Blue":dbl, "Controls"=w509:u8[])  [unwired: 8 in]
            n337 = feedback-in #1(w433) -> ()
            n338 = feedback #2(T6 {"pose"=[0.0, 0.0, 0.0], "totalerror_v"=0.0, "erroSteering"=0.0, "ActualTime"=0.0, "ActualTime 2"=0.0} ("Red feedback init")) -> (w435:T6)
            n339 = call "Controller.vi"("ControllerGains"="ControllerGains Black", "Current State"=w483, "MyID"=w507, "Pose"=w505, "Feedback elements In"=w435, "CurrentWP"=w494, "Vref"=w485, "Trajectory"=w480, "ActualTime"=w506) -> ("Feedback elements Out"=w436:T12, "v_real"=→"Real Speed Black":dbl, "Controls"=w502:u8[])  [unwired: 8 in]
            n340 = feedback-in #2(w436) -> ()
            n341 = feedback #3(T6 {"pose"=[0.0, 0.0, 0.0], "totalerror_v"=0.0, "erroSteering"=0.0, "ActualTime"=0.0, "ActualTime 2"=0.0} ("Red feedback init")) -> (w439:T6)
            n342 = call "Controller.vi"("ControllerGains"="ControllerGains Red", "Current State"=w481, "MyID"=w496, "Pose"=w501, "Feedback elements In"=w439, "CurrentWP"=w493, "Vref"=w487, "Trajectory"=w495, "ActualTime"=w497) -> ("Feedback elements Out"=w440:T12, "v_real"=→"Real Speed Red":dbl, "Controls"=w500:u8[])  [unwired: 8 in]
            n343 = feedback-in #3(w440) -> ()
            n344 = feedback #4(T6 {"pose"=[0.0, 0.0, 0.0], "totalerror_v"=0.0, "erroSteering"=0.0, "ActualTime"=0.0, "ActualTime 2"=0.0} ("Red feedback init")) -> (w474:T6)
            n345 = call "Controller.vi"("ControllerGains"="ControllerGains Grey", "Current State"=w472, "MyID"=w468, "Pose"=w461, "Feedback elements In"=w474, "CurrentWP"=w470, "Vref"=w471, "Trajectory"=w469, "ActualTime"=w463) -> ("Feedback elements Out"=w473:T12, "v_real"=→"Real Speed Grey":dbl, "Controls"=w465:u8[])  [unwired: 8 in]
            n346 = feedback-in #4(w473) -> ()
            n347 = feedback #5(T6 {"pose"=[0.0, 0.0, 0.0], "totalerror_v"=0.0, "erroSteering"=0.0, "ActualTime"=0.0, "ActualTime 2"=0.0} ("Red feedback init")) -> (w443:T6)
            n348 = call "Controller.vi"("ControllerGains"="ControllerGains DarkGrey", "Current State"=w453, "MyID"=w457, "Pose"=w460, "Feedback elements In"=w443, "CurrentWP"=w455, "Vref"=w454, "Trajectory"=w456, "ActualTime"=w459) -> ("Feedback elements Out"=w444:T12, "v_real"=→"Real Speed DarkGrey":dbl, "Controls"=w458:u8[])  [unwired: 8 in]
            n349 = feedback-in #5(w444) -> ()
            n350 = call "CreateSendMSG.vi"("COM Data"=w508, "Controls"=w509) -> ()  [unwired: 18 in]
            n351 = call "CreateSendMSG.vi"("COM Data"=w438, "Controls"=w502) -> ()  [unwired: 18 in]
            n352 = call "CreateSendMSG.vi"("COM Data"=w442, "Controls"=w500) -> ()  [unwired: 18 in]
            n353 = call "CreateSendMSG.vi"("COM Data"=w466, "Controls"=w465) -> ()  [unwired: 18 in]
            n354 = call "CreateSendMSG.vi"("COM Data"=w446, "Controls"=w458) -> ()  [unwired: 18 in]
            n355 = Index Array(array=w509) -> (element #1=→"Blue Steering":u8, element #2=→"Blue Speed":u8)  [unwired: 2 in]
            n356 = Index Array(array=w502) -> (element #1=→"Black Steering":u8, element #2=→"Black Speed":u8)  [unwired: 2 in]
            n357 = Index Array(array=w500) -> (element #1=→"Red Steering":u8, element #2=→"Red Speed":u8)  [unwired: 2 in]
            n358 = Index Array(array=w465) -> (element #1=→"Grey Steering":u8, element #2=→"Grey Speed":u8)  [unwired: 2 in]
            n359 = Index Array(array=w458) -> (element #1=→"DarkGrey Steering":u8, element #2=→"DarkGrey Speed":u8)  [unwired: 2 in]
          }
          frame #6 {
            n360 = local read "Iter"() -> (w517:i32)
            n361 = Quotient & Remainder(x=w517, y=1) -> (x-y*floor(x/y)=w516:i32)  [unwired: 1 out]
            n362 = Equal To 0?(x=w516) -> (x = 0?=w515:bool)
            n363 = local read "Quadcopter"() -> (w512:bool)
            n364 = local read "Visualizer"() -> (w514:bool)
            n365 = And(x=w515, y=w514) -> (x .and. y?=w513:bool)
            n366 = case shown="True" w513 {
              frame False {
              }
              frame True {
                n367 = flat-sequence {
                  frame #0 {
                    n368 = local read "NTrucks"() -> (w556:i32)
                    n369 = Multiply(x=w556, y=3) -> (x*y=w557:i32)
                    n370 = local read "TL Outer Select"() -> (w553:bool)
                    n371 = local read "TL Inner Select"() -> (w554:bool)
                    n372 = local read "Trucks Poses"() -> (w548:dbl[][])
                    n373 = local read "Trailers"() -> (w526:bool[])
                    n374 = global read "Global.vi" "stop"() -> (w547:bool)
                    n375 = Boolean To (0,1)(Boolean=w547) -> (0, 1=w549:i16)
                    n376 = Boolean To (0,1)(Boolean=w553) -> (0, 1=w550:i16)
                    n377 = Boolean To (0,1)(Boolean=w554) -> (0, 1=w551:i16)
                    n378 = Boolean To (0,1)(Boolean=w526) -> (0, 1=w527:i16[])
                    n379 = Reshape Array(w548, w557) -> (w541:dbl[])
                    n380 = local read "Traffic Light Position Outer Lane"() -> (w533:i32)
                    n381 = local read "Traffic Light Position Inner Lane"() -> (w534:i32)
                    n382 = local read "Platooning Distance Scenario"() -> (w532:dbl)
                    n383 = local read "Distance to Master"() -> (w540:dbl[])
                    n384 = local read "StopArrayOuter"() -> (w529:i32[])
                    n385 = local read "StopArrayInner"() -> (w528:i32[])
                    n386 = local read "PlatoonArray"() -> (w530:i32[])
                    n387 = local read "CurrentState"() -> (w537:i32[])
                    n388 = local read "CurrentWP"() -> (w538:i32[])
                    n389 = global read "Global.vi" "RealSpeed"() -> (w536:dbl[])
                    n390 = local read "D2TLFinal"() -> (w539:dbl[])
                    n391 = global read "Global.vi" "MasterID"() -> (w535:i32)
                    n392 = local read "Vref"() -> (w531:dbl[])
                    n393 = Build Array (concatenate)(w549, w550, w551, w533, w534, w535, w532, w536, w537, w538, w539, w540, w531, w530, w529, w528, w527, w541) -> (w552:dbl[])
                    n394 = To Double Precision Float(number=w552) -> (double precision float=w546:dbl[])
                    n395 = Type Cast(x=w546) -> (*(type *) &x=w542:string)  [unwired: 1 in]
                    n396 = local read "Error TCP"() -> (w544:errorcluster)
                    n397 = local read "TCP ID"() -> (w543:refnum<k5>)
                    n398 = TCP Write(connection ID=w543, data in=w542, error in (no error)=w544) -> (error out=w545:errorcluster)  [unwired: 1 in, 2 out]
                    n399 = local write "Error TCP"(w545) -> ()
                  }
                  frame #1 {
                    n400 = local read "ScenarioString"() -> (w560:string)
                    n401 = String Length(string=w560) -> (length=w559:i32)
                    "length" <- w559
                    n402 = To Double Precision Float(number=w559) -> (double precision float=w558:dbl)
                    n403 = Type Cast(x=w558) -> (*(type *) &x=w563:string)  [unwired: 1 in]
                    n404 = local read "Error TCP"() -> (w566:errorcluster)
                    n405 = local read "TCP ID"() -> (w567:refnum<k5>)
                    n406 = TCP Write(connection ID=w567, data in=w563, error in (no error)=w566) -> (connection ID out=w562:refnum<k5>, bytes written=→"bytes written 2":i32, error out=w561:errorcluster)  [unwired: 1 in]
                    n407 = TCP Write(connection ID=w562, data in=w560, error in (no error)=w561) -> (bytes written=→"bytes written 3":i32, error out=w565:errorcluster)  [unwired: 1 in, 1 out]
                    n408 = local write "Error TCP"(w565) -> ()
                  }
                }
              }
            }
            n409 = case shown="True" w512 {
              frame False {
              }
              frame True {
                n410 = global read "Global.vi" "MasterID"() -> (w522:i32)
                n411 = local read "Error TCP_quad"() -> (w524:errorcluster)
                n412 = local read "TCP_quad ID"() -> (w525:refnum<k5>)
                n413 = To Double Precision Float(number=w522) -> (double precision float=w523:dbl)
                n414 = Type Cast(x=w523) -> (*(type *) &x=w521:string)  [unwired: 1 in]
                n415 = TCP Write(connection ID=w525, data in=w521, error in (no error)=w524) -> (connection ID out=w520:refnum<k5>, error out=w519:errorcluster)  [unwired: 1 in, 1 out]
                n416 = local write "TCP_quad ID"(w520) -> ()
                n417 = local write "Error TCP_quad"(w519) -> ()
              }
            }
          }
        }
        n418 = global write "Global.vi" "stop"("stop") -> ()
        n419 = Wait Until Next ms Multiple(millisecond multiple=u32 100) -> ()  [unwired: 1 out]
        "Iter" <- w151
      }
    }
    frame #3 {
      n420 = local read "Visualizer"() -> (w572:bool)
      n421 = local read "Quadcopter"() -> (w569:bool)
      n422 = case shown="True" w569 {
        frame False {
        }
        frame True {
          n423 = local read "Error TCP_quad"() -> (w576:errorcluster)
          n424 = local read "TCP_quad ID"() -> (w577:refnum<k5>)
          n425 = TCP Close Connection(connection ID=w577, error in (no error)=w576) -> ()  [unwired: 1 in, 2 out]
        }
      }
      n426 = case shown="True" w572 {
        frame False {
        }
        frame True {
          n427 = local read "Error TCP"() -> (w587:errorcluster)
          n428 = local read "TCP ID"() -> (w588:refnum<k5>)
          n429 = TCP Close Connection(connection ID=w588, error in (no error)=w587) -> ()  [unwired: 1 in, 2 out]
        }
      }
      n430 = for {
        N: 5 -> [_]
        n431 = local read "COM Blue"() -> (w592:T2)
        n432 = Build Array(u8 127 ("Steering"), u8 127 ("Speed")) -> (w589:u8[])
        n433 = call "CreateSendMSG.vi"("COM Data"=w592, "Controls"=w589) -> ()  [unwired: 18 in]
        n434 = Wait Until Next ms Multiple(millisecond multiple=u32 100) -> ()  [unwired: 1 out]
      }
      n435 = for {
        N: 5 -> [_]
        n436 = local read "COM  Red"() -> (w597:T2)
        n437 = Build Array(u8 127 ("Steering"), u8 127 ("Speed")) -> (w594:u8[])
        n438 = call "CreateSendMSG.vi"("COM Data"=w597, "Controls"=w594) -> ()  [unwired: 18 in]
        n439 = Wait Until Next ms Multiple(millisecond multiple=u32 100) -> ()  [unwired: 1 out]
      }
      n440 = for {
        N: 5 -> [_]
        n441 = local read "COM  Black"() -> (w602:T2)
        n442 = Build Array(u8 127 ("Steering"), u8 127 ("Speed")) -> (w599:u8[])
        n443 = call "CreateSendMSG.vi"("COM Data"=w602, "Controls"=w599) -> ()  [unwired: 18 in]
        n444 = Wait Until Next ms Multiple(millisecond multiple=u32 100) -> ()  [unwired: 1 out]
      }
      n445 = for {
        N: 5 -> [_]
        n446 = local read "COM  Grey"() -> (w585:T2)
        n447 = Build Array(u8 127 ("Steering"), u8 127 ("Speed")) -> (w582:u8[])
        n448 = call "CreateSendMSG.vi"("COM Data"=w585, "Controls"=w582) -> ()  [unwired: 18 in]
        n449 = Wait Until Next ms Multiple(millisecond multiple=u32 100) -> ()  [unwired: 1 out]
      }
      n450 = for {
        N: 5 -> [_]
        (unwired) u32 100 ("millisecond multiple")
        n451 = local read "COM  DarkGrey"() -> (w581:T2)
        n452 = Build Array(u8 127 ("Steering"), u8 127 ("Speed")) -> (w578:u8[])
        n453 = call "CreateSendMSG.vi"("COM Data"=w581, "Controls"=w578) -> ()  [unwired: 18 in]
      }
    }
  }
